vi "Measure Fringe Displacement Simple.vi"(0 "Photodiode Output":dbl, 7 "Fringe Counter Settings":T1={"Wavelength"=6e-07, "Divisions"=2.0, "Scaling Amplitude"=1.2, "Scaling Offset"=0.0} {"Scaling Offset" format="%0.2f"; "Scaling Amplitude" format="%0.2f"}, 9 "Reset":bool) -> (4 "Displacement":dbl=6e-06, 6 "Input Signals":dbl[][](graph), 8 "Stepped Signal":dbl(graph), 10 "Output Signal":dbl[](graph), 15 "Initial Step Position":dbl)   [LabVIEW 2014]
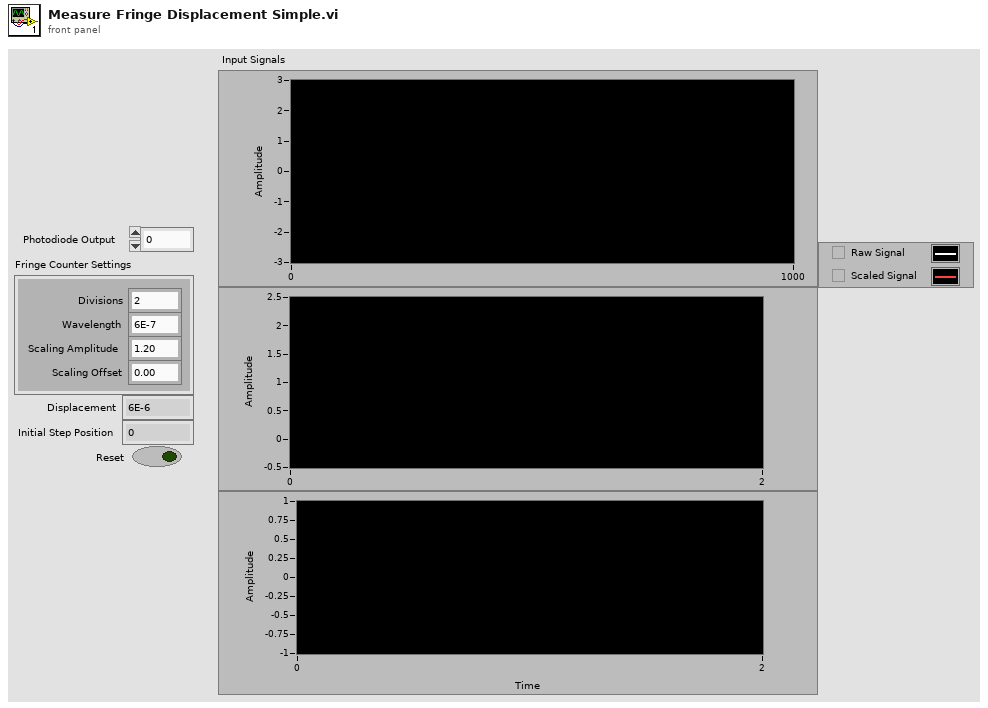
[diagram p1: front panel]
types:
  T1 = cluster{"Wavelength":dbl, "Divisions":dbl, "Scaling Amplitude":dbl, "Scaling Offset":dbl}
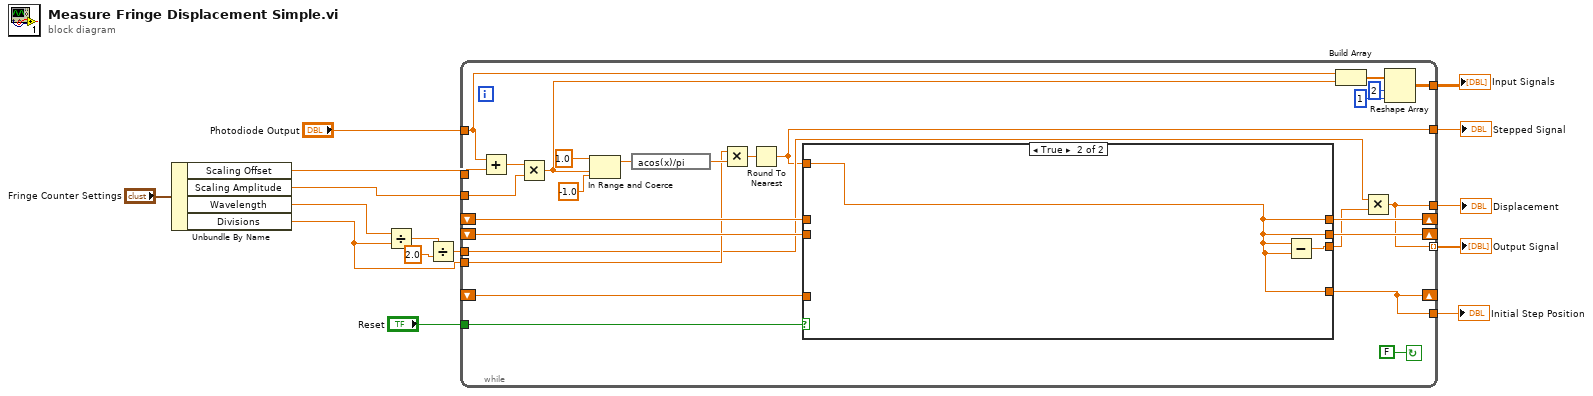
[diagram p0: block diagram]
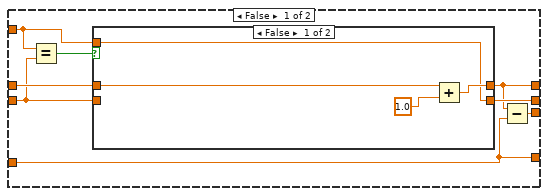
[diagram p2: hidden frame]
diagram:
  n1 = Unbundle By Name("Fringe Counter Settings") -> ("Scaling Offset"=w4:dbl, "Scaling Amplitude"=w3:dbl, "Wavelength"=w2:dbl, "Divisions"=w1:dbl)
  n2 = Divide(x=w2, y=w1) -> (x/y=w6:dbl)
  n3 = Divide(x=w6, y=2.0) -> (x/y=w8:dbl)
  n4 = while {
    tunnel: [w32] -> w10 mode=indexing
    shift-right: [w33] -> _
    shift-left: _ -> [w41]
    shift-right: [w35] -> _
    shift-left: _ -> [w42]
    tunnel: w1 -> [w34]
    tunnel: [w32] -> w9
    tunnel: w8 -> [w31]
    tunnel: w4 -> [w28]
    tunnel: w3 -> [w27]
    tunnel: [w25] -> w11
    tunnel: [w20] -> w12
    tunnel: "Photodiode Output" -> [w19]
    shift-right: [w17] -> _
    shift-left: _ -> [w18]
    tunnel: [w17] -> w14
    tunnel: "Reset" -> [w16]
    stop <- FALSE continue-if-true
    n5 = Add(x=w19, y=w28) -> (x+y=w29:dbl)
    n6 = Multiply(x=w29, y=w27) -> (x*y=w24:dbl)
    n7 = In Range and Coerce(upper limit=1.0, x=w24, lower limit=-1.0) -> (coerced(x)=w38:dbl)  [unwired: 1 out]
    n8 = expression code="acos(x)/pi"(w38) -> (w39:dbl)
    n9 = Multiply(x=w34, y=w39) -> (x*y=w40:dbl)
    n10 = Round To Nearest(number=w40) -> (nearest integer value=w25:dbl)
    n11 = case shown="True" w16 {
      tunnel: w42 -> [w48 _]
      tunnel: w41 -> [w49 _]
      tunnel: w25 -> [w46 w57]
      tunnel: [w47 w57] -> w35
      tunnel: [w44 w57] -> w33
      tunnel: [w45 w58] -> w30
      tunnel: w18 -> [w43 _]
      tunnel: [w43 w57] -> w17
      frame False {
        n12 = Equal?(x=w46, y=w48) -> (x = y?=w50:bool)
        n13 = case shown="False" w50 {
          tunnel: [w54 w56] -> w44
          tunnel: w49 -> [w52 w56]
          tunnel: w48 -> [_ w55]
          tunnel: [w53 w55] -> w47
          tunnel: w46 -> [w53 _]
          frame False {
            n14 = Add(x=w52, y=1.0) -> (x+y=w54:dbl)
          }
          frame True {
          }
        }
        n15 = Subtract(x=w44, y=w43) -> (x-y=w45:dbl)
      }
      frame True {
        n16 = Subtract(x=w57, y=w57) -> (x-y=w58:dbl)
      }
    }
    n17 = Build Array(w19, w24) -> (w23:dbl[])
    n18 = Multiply(x=w31, y=w30) -> (x*y=w32:dbl)
    n19 = Reshape Array(w23, 2 ("dimension size"), 1 ("dimension size")) -> (w20:dbl[][])
  }
  "Output Signal" <- w10
  "Displacement" <- w9
  "Stepped Signal" <- w11
  "Input Signals" <- w12
  "Initial Step Position" <- w14
